vi "Test 7 Cross Within limits.vi"(8 "error in (no error)":errorcluster, 11 "Test Case In":refnum<class "Vector Test.lvclass">) -> (0 "error out":errorcluster, 3 "Test Case Out":refnum<class "Vector Test.lvclass">)   [LabVIEW 2021, in "Vector Test.lvclass"]
uses:
  Vector Test.lvclass
  Vector Test.lvclass/Vector Test.ctl
  Vector/Vector.lvclass
  <vilib>/Astemes/LUnit/Test Case.lvclass
  C:/Program Files (x86)/National Instruments/LabVIEW 2021/vi.lib/Astemes/LUnit/Test Case.lvclass
  C:/Program Files (x86)/National Instruments/LabVIEW 2021/vi.lib/Astemes/LUnit/LUnit Runnable.lvclass
  C:/git/aoc-2023/Day 24/Vector Test/Vector Test.lvclass
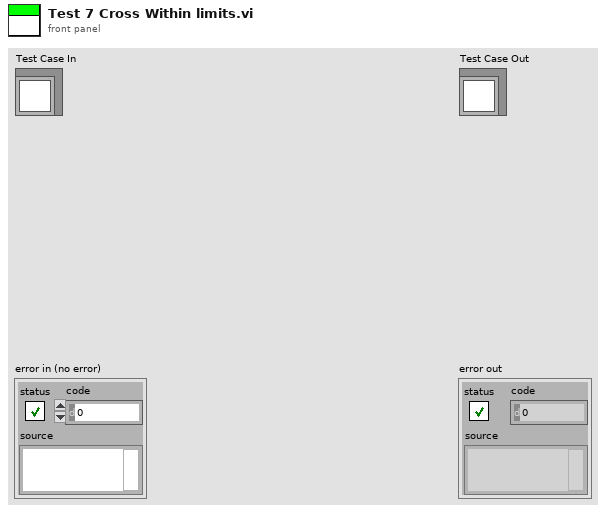
[diagram p1: front panel]
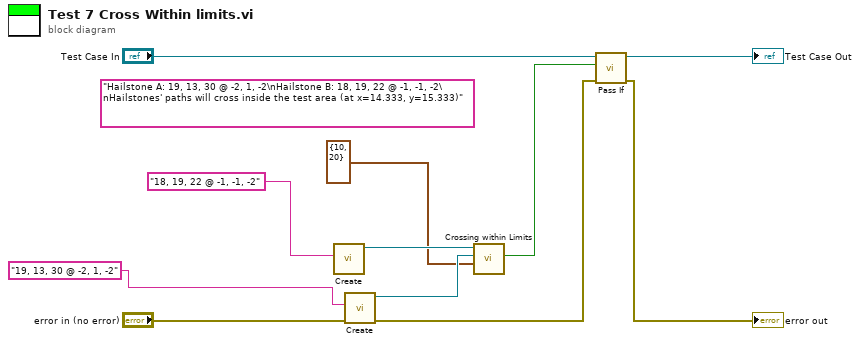
[diagram p0: block diagram]
diagram:
  (unwired) "Hailstone A: 19, 13, 30 @ -2, 1, -2\nHailstone B: 18, 19, 22 @ -1, -1, -2\nHailstones' paths will cross inside the test area (at x=14.333, y=15.333)" ("Input")
  n1 = call "Create.vi"("Input"="18, 19, 22 @ -1, -1, -2") -> ("Hailstone Out"=w5:refnum<class "Vector.lvclass">)  [unwired: 9 in, 1 out]
  n2 = call "Create.vi"("error in (no error)"="error in (no error)", "Input"="19, 13, 30 @ -2, 1, -2") -> ("error out"=w7:errorcluster, "Hailstone Out"=w4:refnum<class "Vector.lvclass">)  [unwired: 8 in]
  n3 = call "Crossing within Limits.vi"("Limits"=cluster{"Min":i64, "Max":i64} {"Min"=10, "Max"=20}, "Vector 2"=w4, "Vector In"=w5) -> ("Crossing within Limits?"=w3:bool)  [unwired: 6 in, 2 out]
  n4 = call <vilib>:"Pass If.vi"("error in (no error)"=w7, "Pass?"=w3, "LUnit Test Case In"="Test Case In") -> ("error out"=→"error out":errorcluster, "LUnit Test Case Out"=→"Test Case Out":refnum<class "Vector Test.lvclass">)  [unwired: 7 in]
